vi "Check Indicator Description.vi"(7 "VolatusAPI":refnum<class "VolatusAPI.lvclass">, 8 "error in (no error)":errorcluster, 10 "Ref":refnum<vi>) -> (0 "error out":errorcluster, 1 "Register":bool, 2 "Indicator":refnum<class "Indicator.lvclass">)   [LabVIEW 2020, in "VolatusGUI.lvlib" / "PluginGUI.lvclass"]
uses:
  PluginGUI.lvclass
  Indicator/Indicator.lvclass
  Volatus/VolatusAPI/VolatusAPI.lvclass
  120e7ead-8603-4b6a-a541-acdea3692ca6.vi
  <vilib>/JDP Science/JSONtext/Next JSON Value.vi
  <vilib>/JDP Science/JSONtext/String Subset.vi
  <vilib>/JDP Science/JSONtext/Parsing/Advance past next JSON Value (inlined COPY).vi
  <vilib>/JDP Science/JSONtext/Parsing/Advance past whitespace.vi
  <vilib>/JDP Science/JSONtext/Parsing/Advance past String.vi
  <vilib>/JDP Science/JSONtext/Parsing/Advance past Number.vi
  <vilib>/JDP Science/JSONtext/Parsing/Advance past Line Ending.vi
  <vilib>/JDP Science/JSONtext/Parsing/Parse Full Path or Item Name.vi
  <vilib>/JDP Science/JSONtext/Parsing/Advance past Array.vi
  <vilib>/JDP Science/JSONtext/Parsing/Advance past Object.vi
  <vilib>/JDP Science/JSONtext/support/Error Cluster From Code.vi
  <vilib>/JDP Science/JSONtext/Offset/Find Item Locations by Path.vi
  <vilib>/JDP Science/JSONtext/JSON text to Variant.vi
  <vilib>/JDP Science/JSONtext/LVClass Serializer/JSONtext LVClass Serializer.lvclass
  PluginGUI.lvclass/PluginGUI.ctl
  <vilib>/JDP Science/JSONtext/JSONtext.lvlib
  VolatusGUI.lvlib
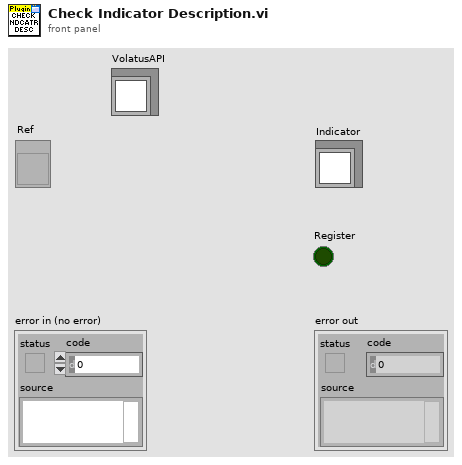
[diagram p1: front panel]
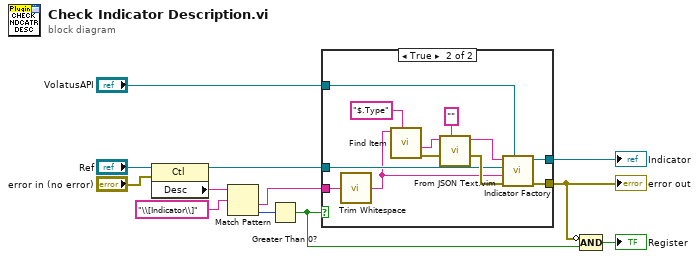
[diagram p0: block diagram]
diagram:
  n1 = property class="Ctl"(reference="Ref", error in="error in (no error)") -> (reference out=w5:refnum<vi>, "Desc"=w10:string)  [unwired: 1 out]
  n2 = Match Pattern(string=w10, regular expression="\\[Indicator\\]") -> (after substring=w6:string, offset past match=w8:i32)  [unwired: 1 in, 2 out]
  n3 = Greater Than 0?(x=w8) -> (x > 0?=w7:bool)
  n4 = case shown="True" w7 {
    tunnel: w6 -> [_ w23]
    tunnel: w5 -> [_ w18]
    tunnel: [_ w15] -> w4
    tunnel: [_ w14] -> w2
    tunnel: "VolatusAPI" -> [_ w13]
    frame False {
    }
    frame True {
      n5 = call <vilib>:"Trim Whitespace.vi"("string"=w23) -> ("trimmed string"=w16:string)  [unwired: 1 in]
      n6 = call <vilib>:"Find Item.vi"("$Path or Item Name"="$.Type", "JSON"=w16) -> ("error out"=w21:errorcluster, "<JSON>"=w20:string)  [unwired: 6 in, 2 out]
      n7 = call "From JSON Text.vim"("Data Type and Default Value"="", "error in (no error)"=w21, "JSON"=w20) -> ("error out"=w24:errorcluster, "Data out"=w17:string)  [unwired: 7 in]
      n8 = call "Indicator Factory.vi"("VolatusAPI"=w13, "error in (no error)"=w24, "JSON"=w16, "Ref"=w18, "Indicator Type"=w17) -> ("error out"=w14:errorcluster, "VolatusGUI:Indicator"=w15:refnum<class "Indicator.lvclass">)  [unwired: 5 in]
    }
  }
  "error out" <- w2
  "Indicator" <- w4
  n9 = Compound Arithmetic op=AND(invert w2, w7) -> (→"Register":bool)
